vi "Write Bool A.vi"(8 "error in (no error)":errorcluster, 10 "Abs_Types.lvlib:Boolean.lvclass":refnum<class "Abs_Boolean.lvclass">, 11 "One Terminal in":refnum<class "AbsFunc_One Term_Bool.lvclass">) -> (0 "error out":errorcluster, 3 "One Terminal out":refnum<class "AbsFunc_One Term_Bool.lvclass">)   [LabVIEW 2021, in "AbsFunc_One Term_Bool.lvclass"]
uses:
  AbsFunc_One Term_Bool.lvclass
  Abs_Types/Boolean/Abs_Boolean.lvclass
  AbsFunc_One Term_Bool.lvclass/AbsFunc_One Term_Bool.ctl
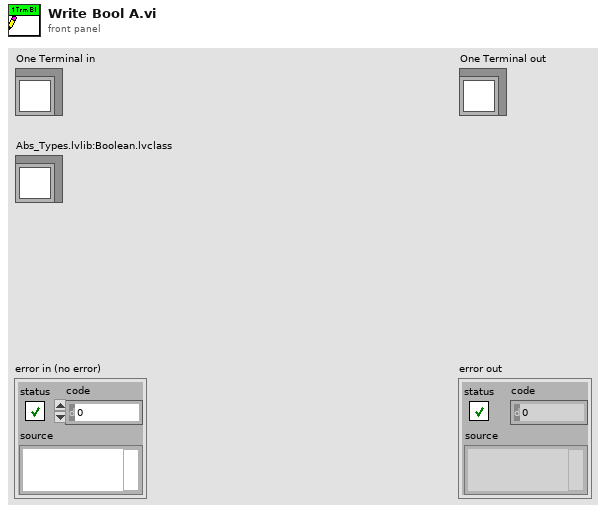
[diagram p1: front panel]
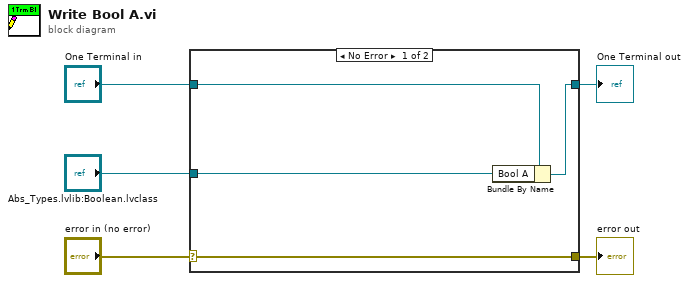
[diagram p0: block diagram]
diagram:
  n1 = case shown="No Error" "error in (no error)" {
    selector: "error in (no error)" -> [w9 w10]
    tunnel: [w9 w10] -> w4
    tunnel: [w7 w11] -> w2
    tunnel: "One Terminal in" -> [w8 w11]
    tunnel: "Abs_Types.lvlib:Boolean.lvclass" -> [w6 _]
    frame No Error {
      n2 = Bundle By Name(cluster=w8, "Bool A"=w6) -> (w7:refnum<class "AbsFunc_One Term_Bool.lvclass">)
    }
    frame Error {
    }
  }
  "error out" <- w4
  "One Terminal out" <- w2
